vi "Convert Temperatures.vi"() -> ()   [LabVIEW 2012]
panel:
  out "温度（绝对温度）":dbl[](array[numeric])
  in  "温度（摄氏度）":dbl[](array[numeric])=[-120.0, -200.0, -75.0, -45.0, -274.0]
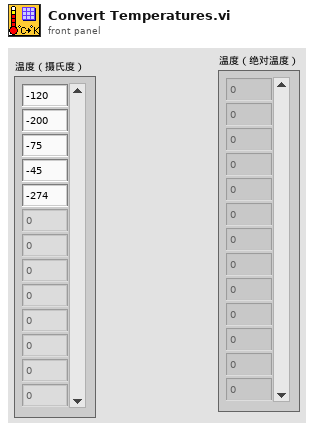
[diagram p1: front panel]
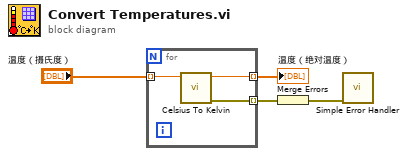
[diagram p0: block diagram]
diagram:
  n1 = for {
    tunnel: "温度（摄氏度）" -> [w7] mode=indexing
    tunnel: [w6] -> w3 mode=indexing
    tunnel: [w5] -> w2 mode=indexing
    n2 = call "Celsius To Kelvin.vi"("摄氏度值"=w7) -> ("错误输出"=w5:cluster{"状态":bool, "代码":i32, "源":string}, "绝对温度值"=w6:dbl)  [unwired: 9 in]
  }
  "温度（绝对温度）" <- w3
  n3 = Merge Errors ("合并错误")(w2) -> (w1:errorcluster)
  n4 = call <vilib>:"Simple Error Handler.vi"("error in (no error)"=w1) -> ()  [unwired: 4 in, 5 out]
